vi "Deadband Joysticks.vi"(6 "Deadband Z":dbl, 7 "X":dbl, 8 "Deadband Y":dbl, 9 "Deadband X":dbl, 10 "Z":dbl, 11 "Y":dbl) -> (1 "Z'":dbl, 2 "Y'":dbl, 3 "X'":dbl)   [LabVIEW 2015]
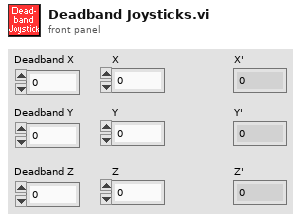
[diagram p1: front panel]
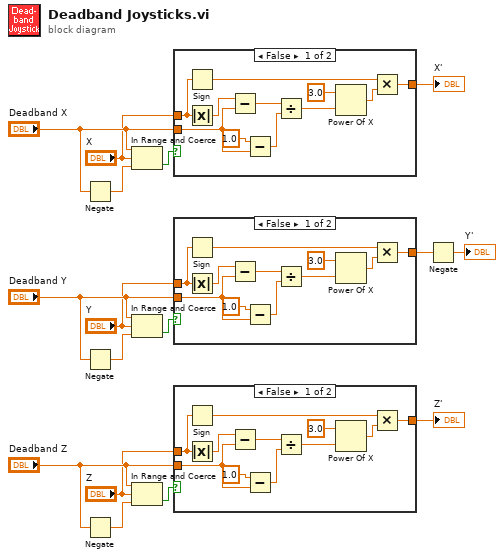
[diagram p0: block diagram]
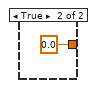
[diagram p2: hidden frame]
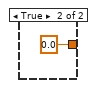
[diagram p3: hidden frame]
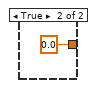
[diagram p4: hidden frame]
diagram:
  n1 = Negate(x="Deadband X") -> (-x=w16:dbl)
  n2 = Negate(x="Deadband Y") -> (-x=w11:dbl)
  n3 = Negate(x="Deadband Z") -> (-x=w7:dbl)
  n4 = In Range and Coerce(upper limit="Deadband X", x="X", lower limit=w16) -> (In Range?=w13:bool)  [unwired: 1 out]
  n5 = In Range and Coerce(upper limit="Deadband Y", x="Y", lower limit=w11) -> (In Range?=w8:bool)  [unwired: 1 out]
  n6 = In Range and Coerce(upper limit="Deadband Z", x="Z", lower limit=w7) -> (In Range?=w4:bool)  [unwired: 1 out]
  n7 = case shown="False" w13 {
    tunnel: "Deadband X" -> [w22 _]
    tunnel: "X" -> [w21 _]
    tunnel: [w20 0.0] -> w12
    frame False {
      n8 = Sign(1:w21) -> (0:w23:dbl)
      n9 = Absolute Value(x=w21) -> (abs(x)=w26:dbl)
      n10 = Subtract(x=w26, y=w22) -> (x-y=w25:dbl)
      n11 = Subtract(x=1.0, y=w22) -> (x-y=w24:dbl)
      n12 = Divide(x=w25, y=w24) -> (x/y=w18:dbl)
      n13 = Power Of X(1:w18, 2:3.0 ("y")) -> (0:w19:dbl)
      n14 = Multiply(x=w23, y=w19) -> (x*y=w20:dbl)
    }
    frame True {
    }
  }
  "X'" <- w12
  n15 = case shown="False" w8 {
    tunnel: "Deadband Y" -> [w34 _]
    tunnel: "Y" -> [w33 _]
    tunnel: [w32 0.0] -> w2
    frame False {
      n16 = Sign(1:w33) -> (0:w35:dbl)
      n17 = Absolute Value(x=w33) -> (abs(x)=w38:dbl)
      n18 = Subtract(x=w38, y=w34) -> (x-y=w37:dbl)
      n19 = Subtract(x=1.0, y=w34) -> (x-y=w36:dbl)
      n20 = Divide(x=w37, y=w36) -> (x/y=w31:dbl)
      n21 = Power Of X(1:w31, 2:3.0 ("y")) -> (0:w30:dbl)
      n22 = Multiply(x=w35, y=w30) -> (x*y=w32:dbl)
    }
    frame True {
    }
  }
  n23 = case shown="False" w4 {
    tunnel: "Deadband Z" -> [w46 _]
    tunnel: "Z" -> [w45 _]
    tunnel: [w44 0.0] -> w3
    frame False {
      n24 = Sign(1:w45) -> (0:w47:dbl)
      n25 = Absolute Value(x=w45) -> (abs(x)=w50:dbl)
      n26 = Subtract(x=w50, y=w46) -> (x-y=w49:dbl)
      n27 = Subtract(x=1.0, y=w46) -> (x-y=w48:dbl)
      n28 = Divide(x=w49, y=w48) -> (x/y=w43:dbl)
      n29 = Power Of X(1:w43, 2:3.0 ("y")) -> (0:w41:dbl)
      n30 = Multiply(x=w47, y=w41) -> (x*y=w44:dbl)
    }
    frame True {
    }
  }
  "Z'" <- w3
  n31 = Negate(x=w2) -> (-x=→"Y'":dbl)
